vi "Write Units.vi"(8 "error in":errorcluster, 10 "Units":T1, 11 "PRM in":refnum<class "PRM.lvclass">) -> (0 "error out":errorcluster, 3 "PRM out":refnum<class "PRM.lvclass">)   [LabVIEW 2019, in "PRM.lvlib" / "PRM.lvclass"]
uses:
  Library/PRM.lvclass
  Custom Controls/Units.ctl
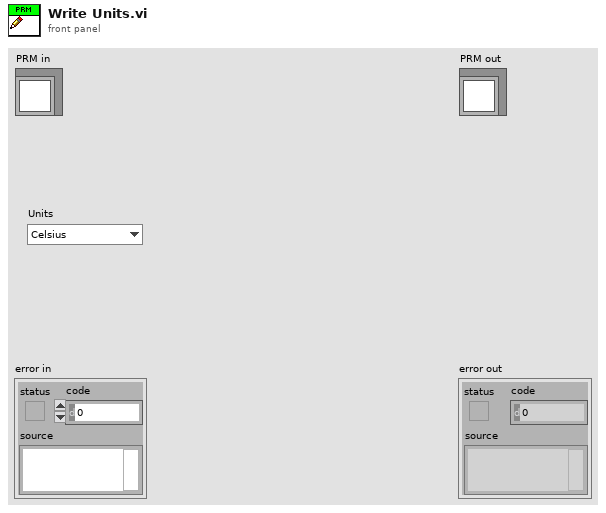
[diagram p1: front panel]
types:
  T1 = typedef "PRM.lvlib/PRM.lvclass/Units.ctl" = enum16{"Celsius", "Fahrenheit", "Kelvin", "Ohms"}
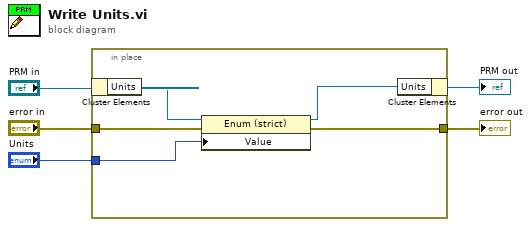
[diagram p0: block diagram]
diagram:
  n1 = in-place {
    in-place-border: "Units" -> [w8]
    in-place-border: "error in" -> [w7]
    in-place-border: [w6] -> w1
    n2 = in-place-cluster #1("PRM in") -> ("Units"=w10:refnum<vi>)
    n3 = property class="Enum (strict)"(reference=w10, error in=w7, "Value"=w8) -> (reference out=w9:refnum<vi>, error out=w6:errorcluster)
    n4 = in-place-cluster #1("Units"=w9) -> (→"PRM out":refnum<class "PRM.lvclass">)
  }
  "error out" <- w1
